vi "WaterDelivery.vi"   [LabVIEW 2014]
uses:
  Scanner/Database/Database.lvclass
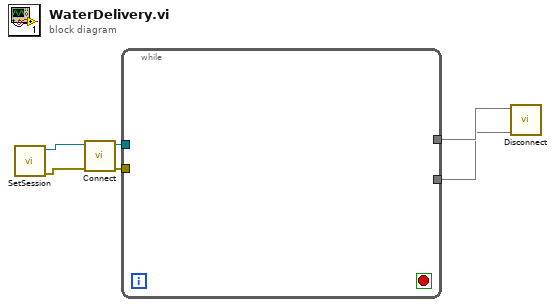
[diagram p0: block diagram]
diagram:
  n1 = call-dynamic "SetSession.vi"() -> ("error out"=w5:errorcluster, "Database out"=w6:refnum<class "Database.lvclass">)  [unwired: 10 in]
  n2 = call-dynamic "Connect.vi"("Database in"=w6, "error in (no error)"=w5) -> ("Database out"=w4:refnum<class "Database.lvclass">, "error out"=w3:errorcluster)  [unwired: 7 in]
  n3 = while {
    tunnel: w4 -> [_]
    tunnel: w3 -> [_]
    tunnel: [_] -> w2
    tunnel: [_] -> w1
    stop <- _ stop-if-true
  }
  n4 = call-dynamic "Disconnect.vi"("error in (no error)"=w1, "Database in"=w2) -> ()  [unwired: 8 in, 2 out]
